vi "Generic Camera Resample Image.vi"(0 "Ref In":T1, 11 "Error In":errorcluster) -> (4 "Ref Out":T1, 15 "Error Out":errorcluster)   [LabVIEW 2020]
uses:
  <vilib>/vision/Image Controls.llb/IMAQ Image.ctl
  Camera Controls/Camera IMAQ Key Info.ctl
  <vilib>/vision/NI_Vision_Development_Module.lvlib
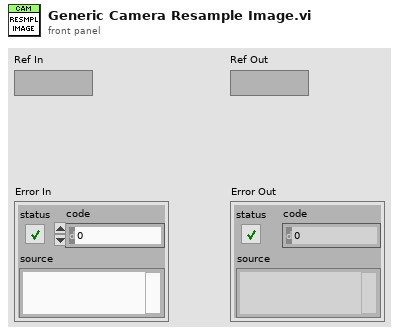
[diagram p1: front panel]
types:
  T1 = typedef "IMAQ Image.ctl" = refnum<image>
  T2 = typedef "Camera IMAQ Key Info.ctl" = cluster{"Frame":u32, "Sensor Height":i32, "Sensor Width":i32, "ROI Height":i32, "ROI Width":i32, "ROI Enable?":bool, "Bit per Pixel":u8, "Binning factor":i32}
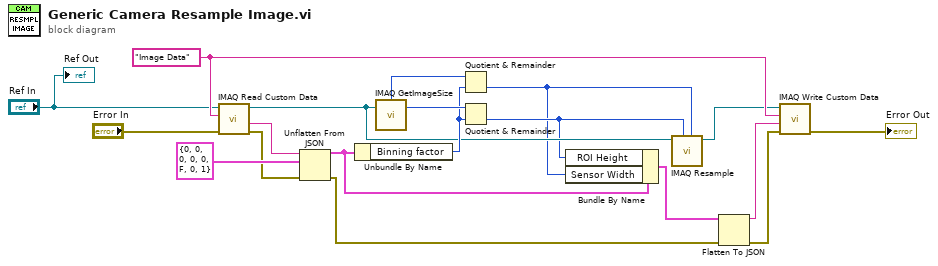
[diagram p0: block diagram]
diagram:
  w16 = "Image Data" ("Key")
  n1 = call "IMAQ Read Custom Data"("error in (no error)"="Error In", "Key"=w16, "Image"="Ref In") -> ("error out"=w15:errorcluster, "Custom Data Out"=w18:string, "Image (duplicate)"=w6:T1)  [unwired: 6 in]
  n2 = Unflatten From JSON(JSON string=w18, type and defaults=T2 {"Frame"=0, "Sensor Height"=0, "Sensor Width"=0, "ROI Height"=0, "ROI Width"=0, "ROI Enable?"=FALSE, "Bit per Pixel"=0, "Binning factor"=1} ("Camera IMAQ Key Info"), error in (no error)=w15) -> (value=w3:T2, error out=w14:errorcluster)  [unwired: 4 in]
  n3 = Unbundle By Name(w3) -> ("Binning factor"=w7:i32)
  n4 = call "IMAQ GetImageSize"("Image"=w6) -> ("Y Resolution"=w8:i32, "X Resolution"=w9:i32)  [unwired: 3 in, 1 out]
  n5 = Quotient & Remainder(x=w9, y=w7) -> (floor(x/y)=w1:i32)  [unwired: 1 out]
  n6 = Quotient & Remainder(x=w8, y=w7) -> (floor(x/y)=w2:i32)  [unwired: 1 out]
  n7 = Bundle By Name(cluster=w3, "ROI Height"=w2, "Sensor Width"=w1) -> (w4:T2)
  n8 = call "IMAQ Resample"("X Resolution"=w1, "Y Resolution"=w2, "Image Src"=w6) -> ("Image Dst Out"=w5:T1)  [unwired: 7 in, 1 out]
  n9 = Flatten To JSON(anything=w4, error in (no error)=w14) -> (JSON string=w17:string, 11:w13:errorcluster)  [unwired: 1 in]
  n10 = call "IMAQ Write Custom Data"("error in (no error)"=w13, "Custom Data In"=w17, "Key"=w16, "Image"=w5) -> ("error out"=→"Error Out":errorcluster)  [unwired: 6 in, 1 out]
  "Ref Out" <- "Ref In"
